vi "Load-lasing-file.vi"(8 "error in (no error)":errorcluster, 11 "Object ref in":T1) -> (0 "error out":errorcluster, 1 "Succes?":bool, 3 "Object ref out":T1)   [LabVIEW 2013, in "SLMControl.lvlib" / "SC-Main.lvclass"]
doc: "Attempts to load an .xml lasing job file from a file drive and send it to the SM1000 device using the .NET API. If the lasing file index is higher than the number of files in the files list, the algorithm starts reiterating again from the beginning of the file list.\n\nThe file is saved to the SM1000 flash memory as 'Tempjob.job'.\n\nOnce sent, the file is loaded as the active job using the TCP API."
uses:
  SC-Main.lvclass
  Object-reference.ctl
  UI/Control-names.ctl
  SC-Main.lvclass/SC-Main.ctl
  Read Lasing control.vi
  Read UI.vi
  UI/Set-control-string.vi
  UI/Set-control-boolean.vi
  SM1000/SM1000.lvclass
  UI/SC-UI.lvclass
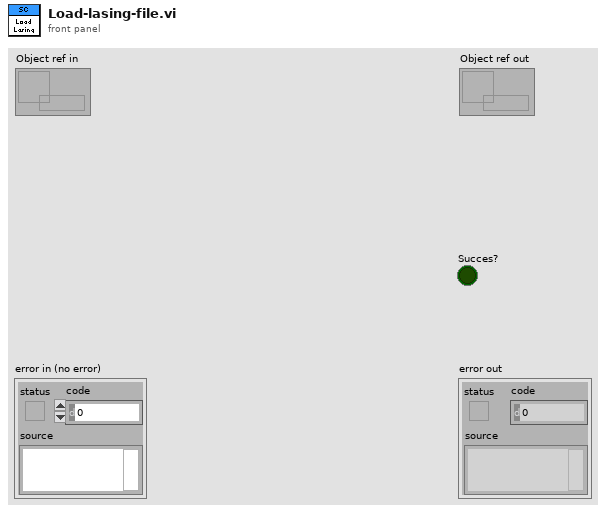
[diagram p1: front panel]
types:
  T1 = typedef "SLMControl.lvlib/SC-Main.lvclass/Object-reference.ctl" = refnum<data-value>
  T2 = typedef "SLMControl.lvlib/SC-UI.lvclass/Control-names.ctl" = enum16{"Com-in", "Com-out", "Help", "Status", "Load configuration", "Save configuration", "Load lasing files", "Load deposition files", "Clear", "Files", "Activate", "Execute", "Abort", "Options", "Current layer", "Current iteration", "Last elapsed time", "Deposition status", "Lasing job", "Status LEDs", "Exiting led", "Initialized led", "Files loaded led", "Activated led", "Executing led", "Deposition led", "Lasing job led", "Lasing led"}
  T3 = typedef "SLMControl.lvlib/SM1000.lvclass/Object-reference.ctl" = refnum<data-value>
  T4 = typedef "SLMControl.lvlib/SC-UI.lvclass/Panes-reference.ctl" = refnum<data-value>
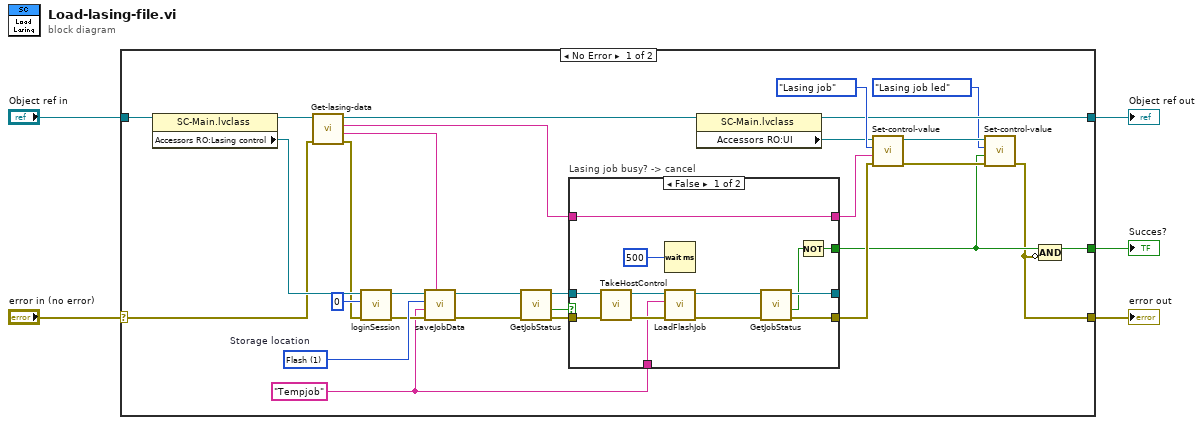
[diagram p0: block diagram]
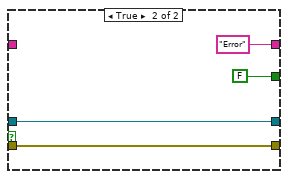
[diagram p2: hidden frame]
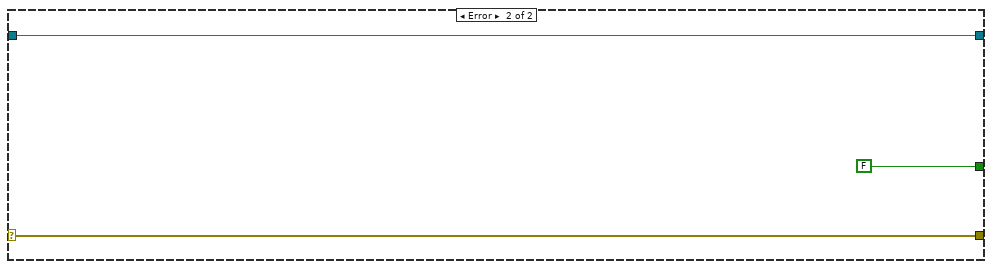
[diagram p3: hidden frame]
diagram:
  n1 = case shown="No Error" "error in (no error)" {
    selector: "error in (no error)" -> [w29 w54]
    tunnel: [w8 w54] -> w4
    tunnel: [w14 w53] -> w2
    tunnel: "Object ref in" -> [w34 w53]
    tunnel: [w9 FALSE] -> w1
    frame No Error {
      w30 = u16 1 items=["Flash"=1, "USB"=2]  # Storage location
      w24 = "Tempjob"
      n2 = property class="SC-Main.lvclass"(reference=w34) -> (reference out=w33:T1, "Accessors RO:Lasing control"=w32:T3)  [unwired: 1 in, 1 out]
      n3 = call "Get-lasing-data.vi"("error in (no error)"=w29, "Object ref in"=w33) -> ("error out"=w28:errorcluster, "Data"=w25:string, "File name"=w19:string, "Object ref out"=w18:T1)  [unwired: 6 in]
      n4 = call "loginSession.vi"("error in (no error)"=w28, "Device index"=0, "SM1000-control in"=w32) -> ("error out"=w26:errorcluster, "SM1000-control out"=w27:T3)  [unwired: 7 in]
      n5 = call "saveJobData.vi"("Job data xml"=w25, "error in (no error)"=w26, "File name wo extension"=w24, "Storage location"=w30, "SM1000-control in"=w27) -> ("error out"=w6:errorcluster, "SM1000-control out"=w7:T3)  [unwired: 5 in]
      n6 = call "GetJobStatus.vi"("error in (no error)"=w6, "SM1000-control in"=w7) -> ("error out"=w23:errorcluster, "Busy?"=w21:bool, "SM1000-control out"=w22:T3)  [unwired: 7 in]
      n7 = case "Lasing job busy? -> cancel" shown="False" w21 {
        tunnel: w24 -> [w45 _]
        tunnel: w23 -> [w44 w49]
        tunnel: w22 -> [w43 w51]
        tunnel: [w41 w51] -> _
        tunnel: [w40 w49] -> w15
        tunnel: [w38 FALSE] -> w10
        tunnel: w19 -> [w37 _]
        tunnel: [w37 "Error" ("t")] -> w16
        frame False {
          n8 = call "TakeHostControl.vi"("error in (no error)"=w44, "SM1000-control in"=w43) -> ("error out"=w46:errorcluster, "SM1000-control out"=w47:T3)  [unwired: 8 in]
          n9 = Wait (ms)(milliseconds to wait=u32 500) -> ()  [unwired: 1 out]
          n10 = call "LoadFlashJob.vi"("error in (no error)"=w46, "Job name wo extension"=w45, "SM1000-control in"=w47) -> ("error out"=w35:errorcluster, "SM1000-control out"=w36:T3)  [unwired: 7 in]
          n11 = call "GetJobStatus.vi"("error in (no error)"=w35, "SM1000-control in"=w36) -> ("error out"=w40:errorcluster, "Busy?"=w39:bool, "SM1000-control out"=w41:T3)  [unwired: 7 in]
          n12 = Not(x=w39) -> (.not. x?=w38:bool)
        }
        frame True {
        }
      }
      n13 = property class="SC-Main.lvclass"(reference=w18) -> (reference out=w14:T1, "Accessors RO:UI"=w17:T4)  [unwired: 1 in, 1 out]
      n14 = call-poly "Set-control-value.vi"("error in (no error)"=w15, "Value"=w16, "Control name"=Control-names."Lasing job", "Panes in"=w17) -> ("error out"=w11:errorcluster, "Panes out"=w13:T4)  [unwired: 6 in]
      n15 = call-poly "Set-control-value.vi"("error in (no error)"=w11, "Value"=w10, "Control name"=Control-names."Lasing job led", "Panes in"=w13) -> ("error out"=w8:errorcluster)  [unwired: 6 in, 1 out]
      n16 = Compound Arithmetic op=AND(w10, invert w8) -> (w9:bool)
    }
    frame Error {
    }
  }
  "error out" <- w4
  "Object ref out" <- w2
  "Succes?" <- w1
